vi "SetConfig.vi"(8 "error in":errorcluster, 10 "S1Config":T1 {"TJHIP_STABLE_CLOSE" format="%#_g sec"; "TJHIP_STABLE_WAIT" format="%#_g sec"; "TJ_PTEST_MAX" format="%#_g in H20"; "TJHIP_TIMER" format="%#_g sec"; "TJLOP_TIMER" format="%#_g sec"; "MSHIP_TIMER" format="%#_g sec"; "S1Z3_LOP_LEAK_MAX" format="%#_g in H20"; "MSLOP_TIMER" format="%#_g sec"; "S1Z3_VENT_PMAX" format="%#_g in H20"}, 11 "Global":T2={"Report Folder Path"=path "", "PT1_MIN"=0.0, "PT1_MAX"=0.0, "VENT_PMAX"=0.0, "LOP_TARGET"=0.0, "LOP_RAMP"=0.0, "LOP_LEAK_MAX"=0.0, "HIP_TARGET"=0.0, "HIP_RAMP"=0.0, "HIP_MIN"=0.0, "HIP_MAX"=0.0, "BLEED_TIME"=0.0, "LOP_MAX"=0.0, "LOP_MIN"=0.0, "PT131Com"="COM5", "PT231Com"="COM6", "PT331Com"="COM7", "PT431Com"="COM8", "PT531Com"="COM9", "PT631Com"="COM10"} {"LOP_MIN" format="%#_g PSI"; "LOP_MAX" format="%#_g PSI"; "BLEED_TIME" format="%#_g Sec"; "HIP_MAX" format="%#_g PSI"; "HIP_MIN" format="%#_g PSI"; "HIP_RAMP" format="%#_g Sec"; "HIP_TARGET" format="%#_g PSI"; "LOP_LEAK_MAX" format="%#_g PSI"; "LOP_RAMP" format="%#_g Sec"; "LOP_TARGET" format="%#_g PSI"; "VENT_PMAX" format="%#_g PSI"; "PT1_MAX" format="%#_g PSI"; "PT1_MIN" format="%#_g PSI"}) -> (0 "error out":errorcluster)   [LabVIEW 2018, in "S1.lvclass"]
uses:
  S1.lvclass
  Controller/Public Controls/GlobalConfig.ctl
  Controller/Public Controls/S1Config.ctl
  Queue/Queue Data.ctl
  Queue/State.ctl
  Controller/GUI.lvclass
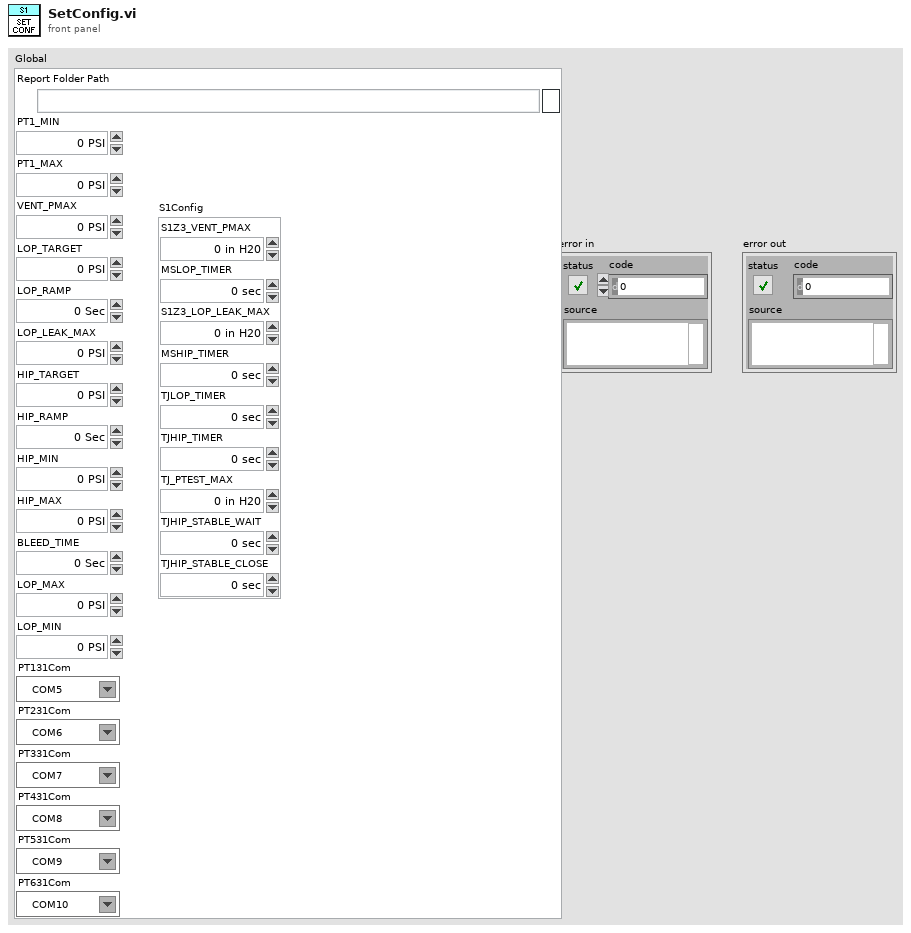
[diagram p1: front panel]
types:
  T1 = typedef "GUI.lvclass/S1Config.ctl" = cluster{"S1Z3_VENT_PMAX":dbl, "MSLOP_TIMER":dbl, "S1Z3_LOP_LEAK_MAX":dbl, "MSHIP_TIMER":dbl, "TJLOP_TIMER":dbl, "TJHIP_TIMER":dbl, "TJ_PTEST_MAX":dbl, "TJHIP_STABLE_WAIT":dbl, "TJHIP_STABLE_CLOSE":dbl}
  T2 = typedef "GUI.lvclass/GlobalConfig.ctl" = cluster{"Report Folder Path":path, "PT1_MIN":dbl, "PT1_MAX":dbl, "VENT_PMAX":dbl, "LOP_TARGET":dbl, "LOP_RAMP":dbl, "LOP_LEAK_MAX":dbl, "HIP_TARGET":dbl, "HIP_RAMP":dbl, "HIP_MIN":dbl, "HIP_MAX":dbl, "BLEED_TIME":dbl, "LOP_MAX":dbl, "LOP_MIN":dbl, "PT131Com":refnum<visa-resource-name>, "PT231Com":refnum<visa-resource-name>, "PT331Com":refnum<visa-resource-name>, "PT431Com":refnum<visa-resource-name>, "PT531Com":refnum<visa-resource-name>, "PT631Com":refnum<visa-resource-name>}
  T3 = typedef "S1.lvclass/Queue Data.ctl" = cluster{"State":T4, "Data":variant}
  T4 = typedef "S1.lvclass/State.ctl" = enum16{"Initialize", "SetConfig", "AckAlarm", "Alarm", "Idle", "LockLid", "LowPressure", "HighPressure", "Vent", "Abort", "Start", "CreateReports", "WriteToReport", "WritePressure", "Error", "Exit"}
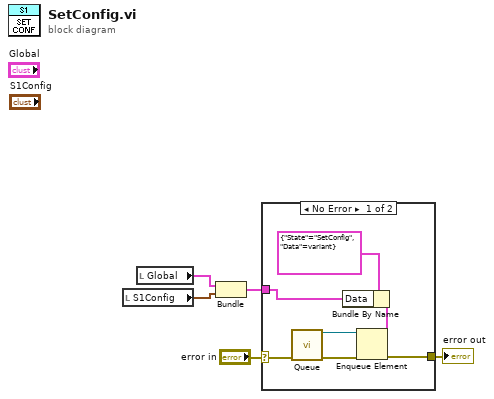
[diagram p0: block diagram]
diagram:
  n1 = local read "S1Config"() -> (w2:T1)
  n2 = local read "Global"() -> (w3:T2)
  n3 = Bundle("Global"=w3, "S1Config"=w2) -> (w1:cluster{"Global":T2, "S1Config":T1})  [unwired: 1 in]
  n4 = case shown="No Error" "error in" {
    selector: "error in" -> [w12 w13]
    tunnel: [w9 w13] -> w5
    tunnel: w1 -> [w6 _]
    frame No Error {
      n5 = call "Queue.vi"("error in"=w12) -> ("error out"=w11:errorcluster, "queue out"=w10:refnum<queue>)  [unwired: 9 in]
      n6 = Bundle By Name(cluster=T3 {"State"=enum."SetConfig", "Data"=variant} ("element"), "Data"=w6) -> (w7:T3)
      n7 = Enqueue Element(queue=w10, element=w7, error in (no error)=w11) -> (error out=w9:errorcluster)  [unwired: 1 in, 2 out]
    }
    frame Error {
    }
  }
  "error out" <- w5
